vi "M05 Hydraulic cells.vi"(11 "EV3 in":T1) -> (3 "EV3 out":T1)   [LabVIEW 2016]
uses:
  <vilib>/NXT/Subs/LVHSConnector.ctl
  <vilib>/NXT/LegoClasses/BrickReference/BrickReference.lvclass
  <vilib>/NXT/Dual Mode Library/Waits/Wait_Num.vi
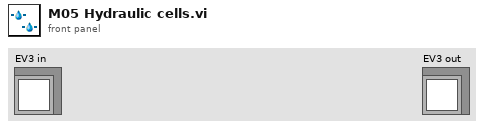
[diagram p1: front panel]
types:
  T1 = typedef "LVHSConnector.ctl" = refnum<class "BrickReference.lvclass">
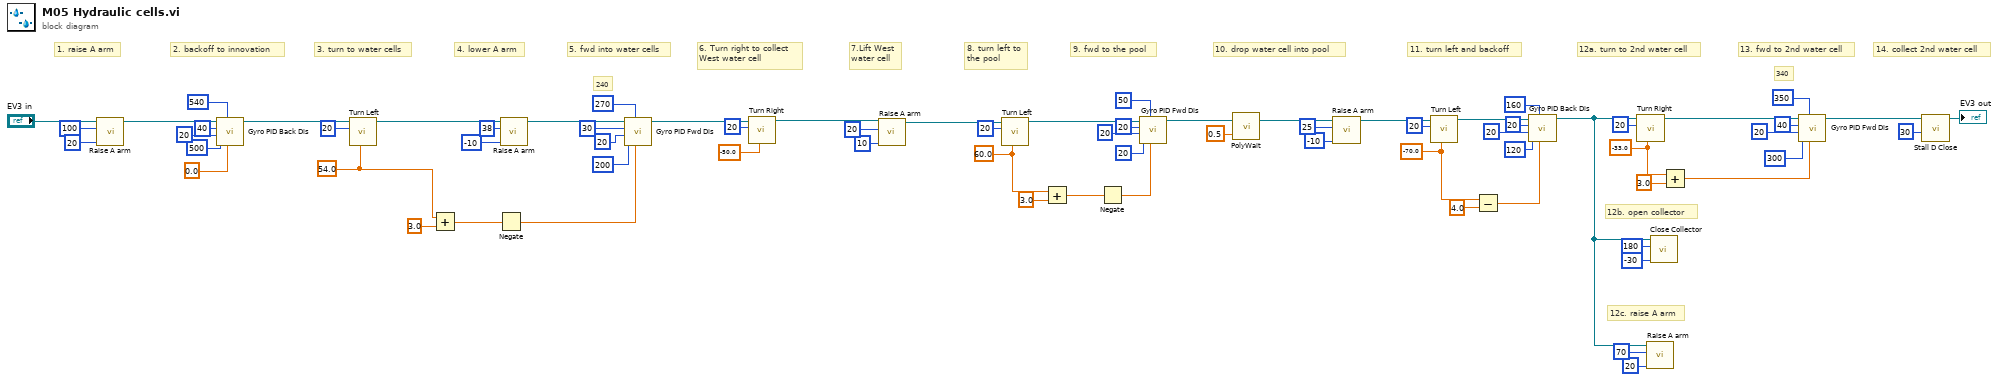
[diagram p0: block diagram]
diagram:
  w4 = sgl -33.0 ("Turning angle")
  w7 = sgl -70.0 ("Turning angle")
  w11 = sgl 60.0 ("Turning angle")
  w53 = sgl 54.0 ("Turning angle")
  # "340"
  # "240"
  # "14. collect 2nd water cell"
  # "13. fwd to 2nd water cell"
  # "12c. raise A arm"
  # "12b. open collector"
  # "12a. turn to 2nd water cell"
  # "11. turn left and backoff"
  # "10. drop water cell into pool"
  # "9. fwd to the pool"
  # "8. turn left to\nthe pool"
  # "7.Lift West\nwater cell"
  # "6. Turn right to collect\nWest water cell"
  # "5. fwd into water cells"
  # "4. lower A arm"
  # "3. turn to water cells"
  # "2. backoff to innovation"
  # "1. raise A arm"
  n1 = call "Raise A arm.vi"("Power"=i8 20, "Rotation"=100, "EV3 in"="EV3 in") -> ("EV3 out"=w69:T1)  [unwired: 8 in]
  n2 = call "Gyro PID Back Dis.vi"("Target angle"=sgl 0.0, "Threshold to stop"=540 ("Threshold to Color"), "Threshold to slow"=500, "Min. speed"=20, "Max. speed"=40, "EV3 in"=w69) -> ("EV3 out"=w63:T1)  [unwired: 5 in]
  n3 = call "Turn Left.vi"("Turning angle"=w53, "Motor B (right)"=i8 20, "EV3 in"=w63) -> ("EV3 out"=w56:T1)  [unwired: 8 in]
  n4 = Add(x=w53, y=sgl 3.0) -> (x+y=w51:sgl)
  n5 = Negate(x=w51) -> (-x=w50:sgl)
  n6 = call "Raise A arm.vi"("Power"=i8 -10, "Rotation"=38, "EV3 in"=w56) -> ("EV3 out"=w54:T1)  [unwired: 8 in]
  n7 = call "Gyro PID Fwd Dis.vi"("Target angle"=w50, "Threshold to stop"=270, "Threshold to slow"=200, "Min. speed"=20, "Max. speed"=30, "EV3 in"=w54) -> ("EV3 out"=w49:T1)  [unwired: 5 in]
  n8 = call "Turn Right.vi"("Turning angle"=sgl -50.0, "Motor B (right)"=i8 20, "EV3 in"=w49) -> ("EV3 out"=w46:T1)  [unwired: 8 in]
  n9 = call "Raise A arm.vi"("Power"=i8 10, "Rotation"=20, "EV3 in"=w46) -> ("EV3 out"=w43:T1)  [unwired: 8 in]
  n10 = call "Turn Left.vi"("Turning angle"=w11, "Motor B (right)"=i8 20, "EV3 in"=w43) -> ("EV3 out"=w41:T1)  [unwired: 8 in]
  n11 = Add(x=w11, y=sgl 3.0) -> (x+y=w9:sgl)
  n12 = Negate(x=w9) -> (-x=w1:sgl)
  n13 = call "Gyro PID Fwd Dis.vi"("Target angle"=w1, "Threshold to stop"=50, "Threshold to slow"=20, "Min. speed"=20, "Max. speed"=20, "EV3 in"=w41) -> ("EV3 out"=w34:T1)  [unwired: 5 in]
  n14 = call-poly <vilib>:"PolyWait.vi"("Time (1 sec)"=sgl 0.5, "NXT/EV3"=w34) -> ("NXT/EV3"=w21:T1)  [unwired: 2 in]
  n15 = call "Raise A arm.vi"("Power"=i8 -10, "Rotation"=25, "EV3 in"=w21) -> ("EV3 out"=w33:T1)  [unwired: 8 in]
  n16 = call "Turn Left.vi"("Turning angle"=w7, "Motor B (right)"=i8 20, "EV3 in"=w33) -> ("EV3 out"=w18:T1)  [unwired: 8 in]
  n17 = Subtract(x=w7, y=sgl 4.0) -> (x-y=w6:sgl)
  n18 = call "Gyro PID Back Dis.vi"("Target angle"=w6, "Threshold to stop"=160, "Threshold to slow"=120, "Min. speed"=20, "Max. speed"=20, "EV3 in"=w18) -> ("EV3 out"=w14:T1)  [unwired: 5 in]
  n19 = call "Turn Right.vi"("Turning angle"=w4, "Motor B (right)"=i8 20, "EV3 in"=w14) -> ("EV3 out"=w22:T1)  [unwired: 8 in]
  n20 = call "Raise A arm.vi"("Power"=i8 20, "Rotation"=70, "EV3 in"=w14) -> ()  [unwired: 8 in, 1 out]
  n21 = call "Close Collector.vi"("Power"=i8 -30, "Rotation"=180, "EV3 in"=w14) -> ()  [unwired: 8 in, 1 out]
  n22 = Add(x=w4, y=sgl 3.0) -> (x+y=w3:sgl)
  n23 = call "Gyro PID Fwd Dis.vi"("Target angle"=w3, "Threshold to stop"=350, "Threshold to slow"=300, "Min. speed"=20, "Max. speed"=40, "EV3 in"=w22) -> ("EV3 out"=w13:T1)  [unwired: 5 in]
  n24 = call "Stall D Close.vi"("Power"=i8 30, "NXT/EV3"=w13) -> ("NXT/EV3"=→"EV3 out":T1)  [unwired: 9 in]
